vi "simulate camera image.vi"(8 "error in (no error)":errorcluster, 11 "FakeCamera in":refnum<class "Point Grey Camera.lvclass">) -> (0 "error out":errorcluster, 2 "Acquisition OK?":bool, 3 "FakeCamera out":refnum<class "Point Grey Camera.lvclass">, 5 "acq time (ms)":u32)   [LabVIEW 2020, in "Point Grey Camera.lvclass"]
uses:
  Point Grey Camera.lvclass
  Point Grey Camera.lvclass/Point Grey Camera.ctl
  NI_Vision_Development_Module.lvlib
panel:
  in  "dont flip":bool
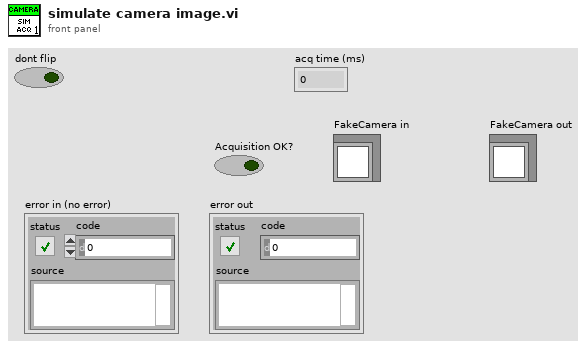
[diagram p1: front panel]
types:
  T1 = typedef "IMAQ Image.ctl" = refnum<image>
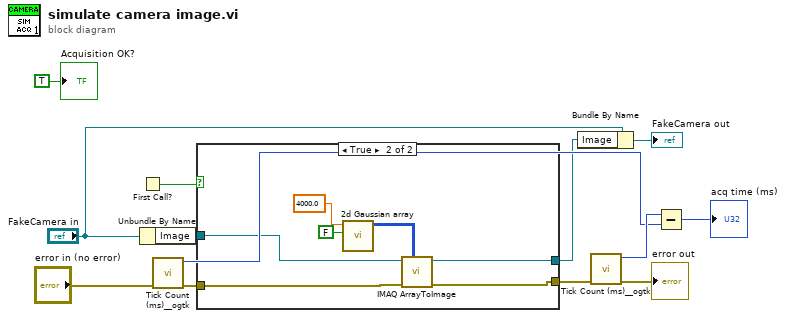
[diagram p0: block diagram]
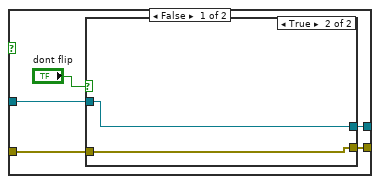
[diagram p2: hidden frame]
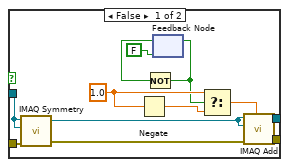
[diagram p3: hidden frame]
diagram:
  n1 = First Call?() -> (First Call?: T/F=w1:bool)
  n2 = Unbundle By Name("FakeCamera in") -> ("Image"=w5:T1)
  n3 = call "Tick Count (ms)__ogtk.vi"("error in (no error)"="error in (no error)") -> ("error out"=w7:errorcluster, "millisecond timer value"=w9:u32)  [unwired: 9 in]
  n4 = case shown="True" w1 {
    tunnel: w7 -> [w17 w39]
    tunnel: [w15 w38] -> w12
    tunnel: [w16 w37] -> w4
    tunnel: w5 -> [w18 w36]
    frame False {
      n5 = case shown="True" "dont flip" {
        tunnel: w18 -> [w30 w32]
        tunnel: w17 -> [w29 w31]
        tunnel: [w21 w32] -> w16
        tunnel: [w20 w31] -> w15
        frame False {
          w25 = 1.0 ("Constant")
          n6 = call "IMAQ Symmetry"("error in (no error)"=w29, "Image Dst"=w30, "Image Src"=w30) -> ("error out"=w19:errorcluster, "Image Dst Out"=w28:T1)  [unwired: 2 in]
          n7 = Negate(x=w25) -> (-x=w24:dbl)
          n8 = feedback #1(FALSE) -> (w27:bool)
          n9 = Not(x=w27) -> (.not. x?=w23:bool)
          n10 = feedback-in #1(w23) -> ()
          n11 = Select(t=w25, s=w23, f=w24) -> (s? t:f=w22:dbl)
          n12 = call "IMAQ Add"("Image Src A"=w28, "Constant"=w22, "Image Dst"=w28, "error in (no error)"=w19) -> ("Image Dst Out"=w21:T1, "error out"=w20:errorcluster)  [unwired: 3 in]
        }
        frame True {
        }
      }
    }
    frame True {
      n13 = call "2d Gaussian array.vi"("multiply A by random number"=FALSE, "A"=4000.0) -> ("Intensity Graph"=w35:u16[][])  [unwired: 9 in]
      n14 = call "IMAQ ArrayToImage"("Image Pixels (U16)"=w35, "error in (no error)"=w39, "Image"=w36) -> ("error out"=w38:errorcluster, "Image Out"=w37:T1)  [unwired: 7 in]
    }
  }
  n15 = Bundle By Name(cluster="FakeCamera in", "Image"=w4) -> (→"FakeCamera out":refnum<class "Point Grey Camera.lvclass">)
  n16 = call "Tick Count (ms)__ogtk.vi"("error in (no error)"=w12) -> ("error out"=→"error out":errorcluster, "millisecond timer value"=w10:u32)  [unwired: 9 in]
  n17 = Subtract(x=w10, y=w9) -> (x-y=→"acq time (ms)":u32)
  "Acquisition OK?" <- TRUE ("Acquisition OK?")
